vi "Sub 2.vi"(8 "error in (no error)":errorcluster, 11 "data value reference":refnum<data-value>) -> (0 "error out":errorcluster, 3 "data value reference out":refnum<data-value>)   [LabVIEW 2009]
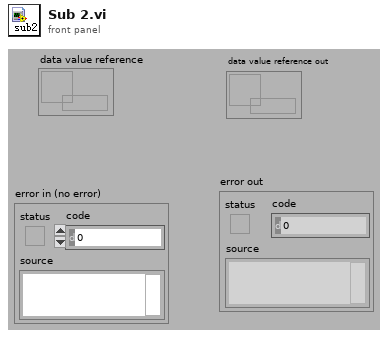
[diagram p1: front panel]
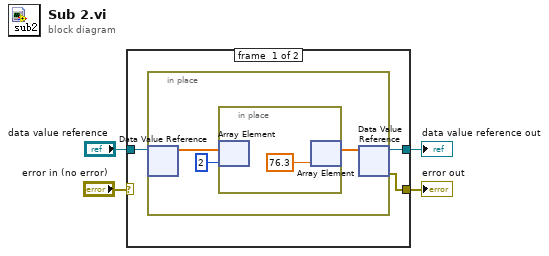
[diagram p0: block diagram]
diagram:
  n1 = case shown="No Error" "error in (no error)" {
    selector: "error in (no error)" -> [_ w12]
    tunnel: "data value reference" -> [w7 w13]
    tunnel: [w6 w13] -> w3
    tunnel: [w5 w12] -> w2
    frame #0 {
      n2 = in-place {
        n3 = in-place-dvr #1(w7) -> (w10:dbl[])  [unwired: 1 out]
        n4 = in-place {
          n5 = in-place-array #2(w10, 2) -> ()  [unwired: 1 out]
          n6 = in-place-array #2(76.3 ("element")) -> (w8:dbl[])  [unwired: 1 out]
        }
        n7 = in-place-dvr #1(w8) -> (w6:refnum<data-value>, w5:errorcluster)
      }
    }
    frame #1 {
    }
  }
  "error out" <- w2
  "data value reference out" <- w3
